vi "FFT滤波无mat程序版.vi"(1 "工频频率":dbl, 2 "样本大小":dbl, 3 "时域波形图":waveform(dbl)[](graph)) -> (0 "时域波形图 2":waveform(dbl)[](graph))   [LabVIEW 2014]
uses:
  <vilib>/Analysis/2dsp.llb/Real FFT.vi
  <vilib>/Analysis/2dsp.llb/Inverse Real FFT.vi
  <vilib>/express/express analysis/Spectral/Block/exnSpectralBlock spectral measurements peak poly.vi
  <vilib>/express/express analysis/Spectral/Block/exnSpectralBlock spectral measurements peak WFM.vi
  <vilib>/express/express analysis/Spectral/XNode/ExpressSpectralMeasurementsBlockNode.xnode
  <vilib>/Analysis/NI_AALPro.lvlib
panel:
  out "时域波形图 3":cluster{"f0":dbl, "df":dbl, "magnitude":dbl[]}(graph)
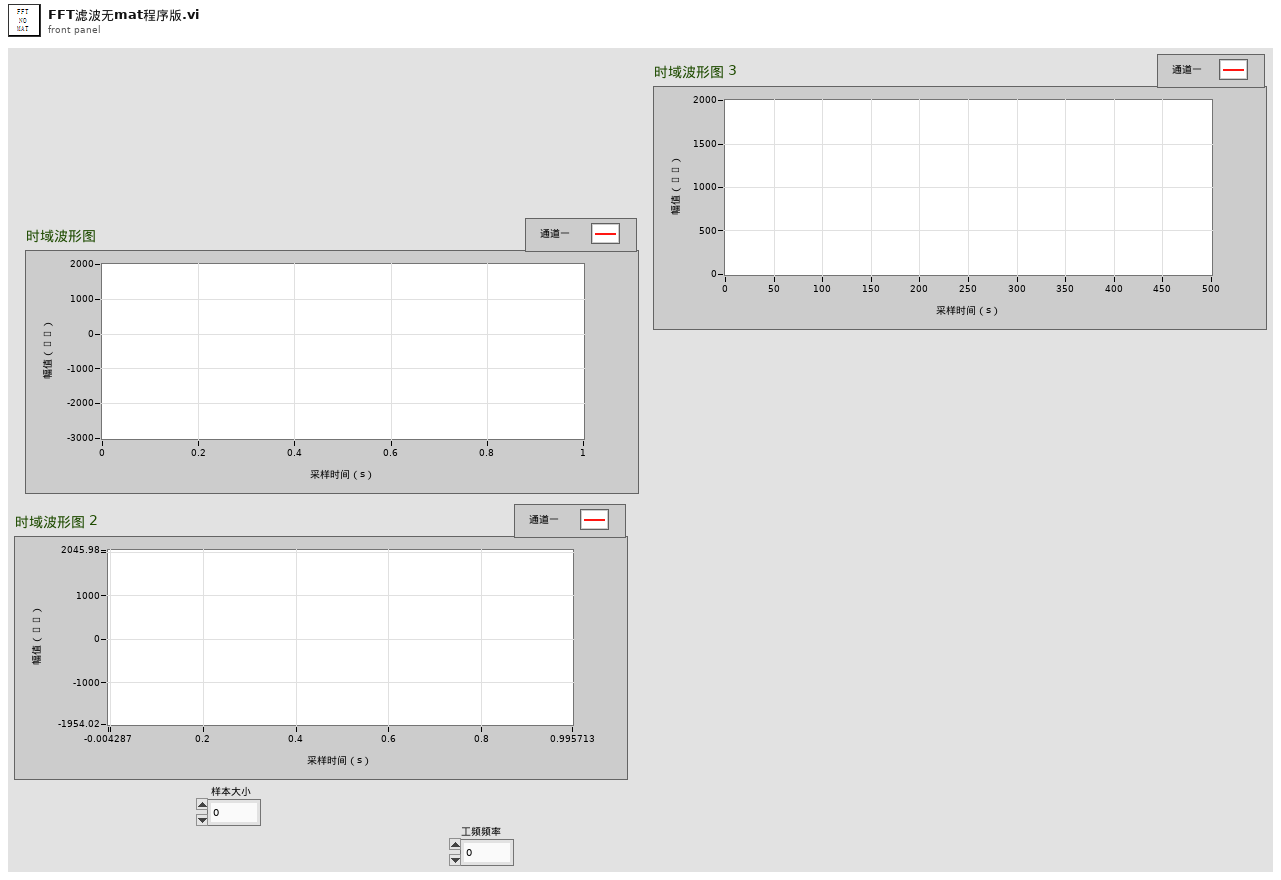
[diagram p1: front panel]
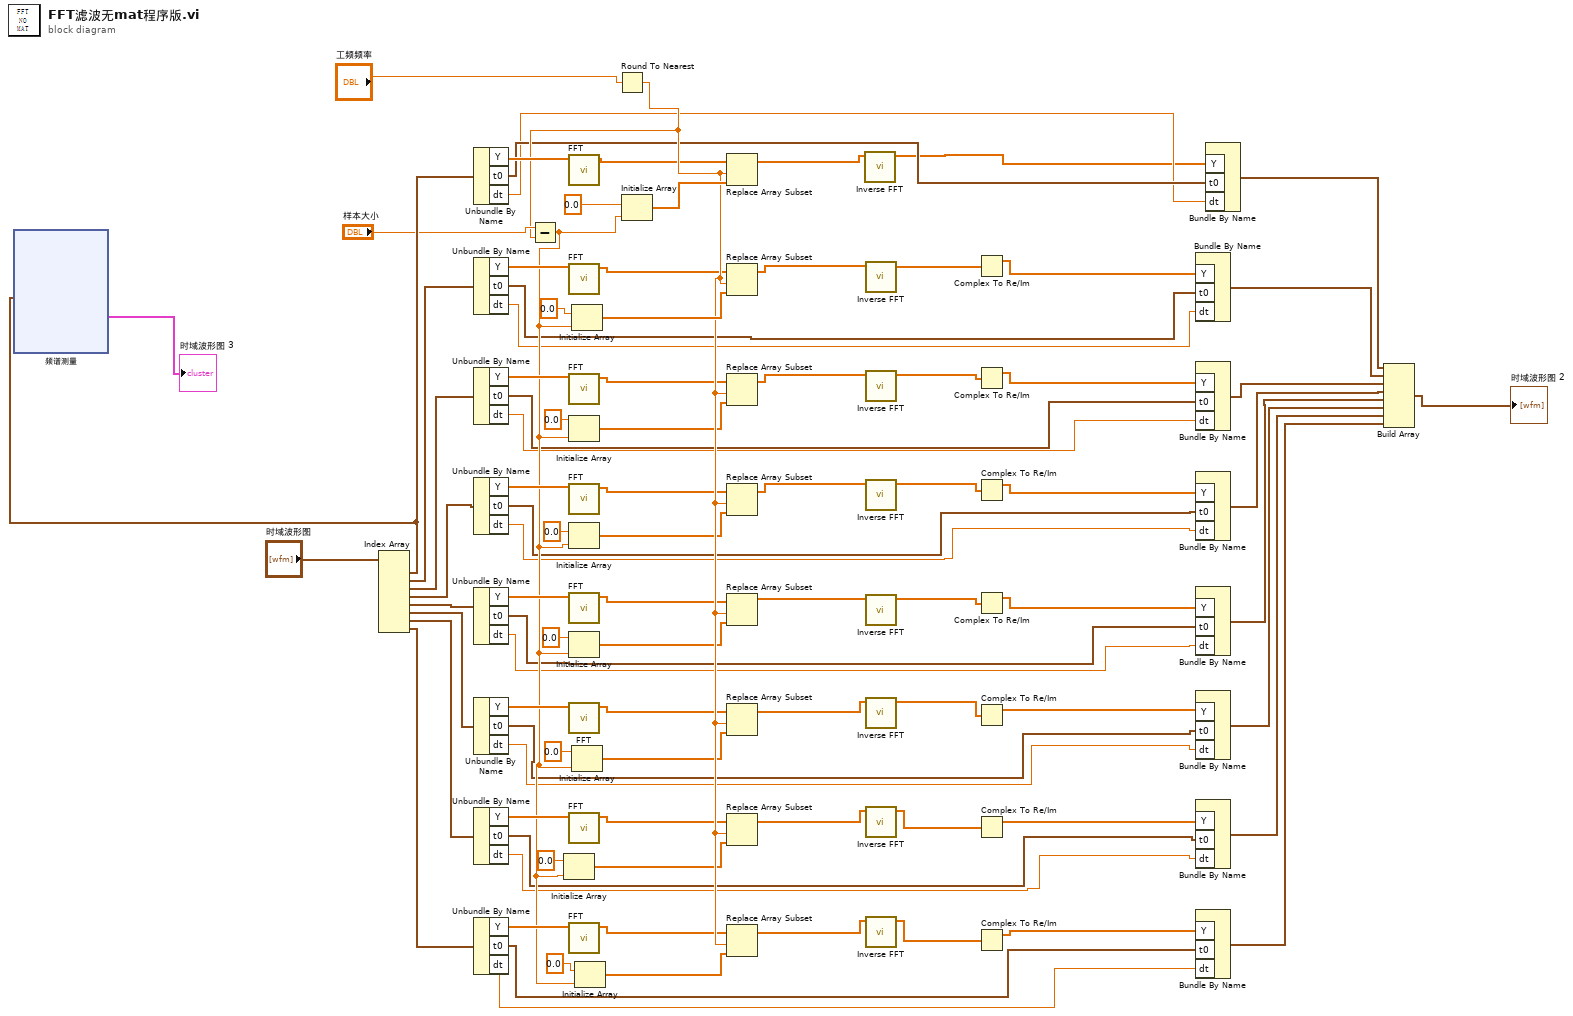
[diagram p0: block diagram]
diagram:
  n1 = Index Array(array="时域波形图") -> (element #1=w70:waveform(dbl), element #2=w93:waveform(dbl), element #3=w92:waveform(dbl), element #4=w91:waveform(dbl), element #5=w90:waveform(dbl), element #6=w89:waveform(dbl), element #7=w88:waveform(dbl), element #8=w87:waveform(dbl))  [unwired: 8 in]
  n2 = xnode "频谱测量"("信号"=w70) -> ("FFT - （峰值）"=→"时域波形图 3":cluster{"f0":dbl, "df":dbl, "magnitude":dbl[]})  [unwired: 1 in, 2 out]
  n3 = Unbundle By Name(w70) -> ("Y"=w86:dbl[], "t0"=w27:timestamp, "dt"=w26:dbl)
  n4 = Unbundle By Name(w93) -> ("Y"=w84:dbl[], "t0"=w25:timestamp, "dt"=w24:dbl)
  n5 = Unbundle By Name(w92) -> ("Y"=w83:dbl[], "t0"=w23:timestamp, "dt"=w22:dbl)
  n6 = Unbundle By Name(w91) -> ("Y"=w82:dbl[], "t0"=w21:timestamp, "dt"=w20:dbl)
  n7 = Unbundle By Name(w90) -> ("Y"=w81:dbl[], "t0"=w19:timestamp, "dt"=w18:dbl)
  n8 = Unbundle By Name(w89) -> ("Y"=w80:dbl[], "t0"=w17:timestamp, "dt"=w16:dbl)
  n9 = Unbundle By Name(w88) -> ("Y"=w79:dbl[], "t0"=w14:timestamp, "dt"=w13:dbl)
  n10 = Unbundle By Name(w87) -> ("Y"=w85:dbl[], "t0"=w12:timestamp, "dt"=w11:dbl)
  n11 = call-poly <vilib>:"FFT.vi"("X"=w86) -> ("FFT {X}"=w10:cdb[])  [unwired: 9 in, 1 out]
  n12 = call-poly <vilib>:"FFT.vi"("X"=w84) -> ("FFT {X}"=w9:cdb[])  [unwired: 9 in, 1 out]
  n13 = call-poly <vilib>:"FFT.vi"("X"=w83) -> ("FFT {X}"=w7:cdb[])  [unwired: 9 in, 1 out]
  n14 = call-poly <vilib>:"FFT.vi"("X"=w82) -> ("FFT {X}"=w6:cdb[])  [unwired: 9 in, 1 out]
  n15 = call-poly <vilib>:"FFT.vi"("X"=w81) -> ("FFT {X}"=w5:cdb[])  [unwired: 9 in, 1 out]
  n16 = call-poly <vilib>:"FFT.vi"("X"=w80) -> ("FFT {X}"=w4:cdb[])  [unwired: 9 in, 1 out]
  n17 = call-poly <vilib>:"FFT.vi"("X"=w79) -> ("FFT {X}"=w3:cdb[])  [unwired: 9 in, 1 out]
  n18 = call-poly <vilib>:"FFT.vi"("X"=w85) -> ("FFT {X}"=w2:cdb[])  [unwired: 9 in, 1 out]
  n19 = Round To Nearest(number="工频频率") -> (nearest integer value=w55:dbl)
  n20 = Subtract(x="样本大小", y=w55) -> (x-y=w57:dbl)
  n21 = Initialize Array(0.0, w57) -> (w50:dbl[])
  n22 = Initialize Array(0.0, w57) -> (w54:dbl[])
  n23 = Initialize Array(0.0, w57) -> (w53:dbl[])
  n24 = Initialize Array(0.0, w57) -> (w52:dbl[])
  n25 = Initialize Array(0.0, w57) -> (w56:dbl[])
  n26 = Initialize Array(0.0, w57) -> (w51:dbl[])
  n27 = Initialize Array(0.0, w57) -> (w49:dbl[])
  n28 = Initialize Array(0.0, w57) -> (w67:dbl[])
  n29 = Replace Array Subset(array=w10, new element=w67, index=w55) -> (w65:cdb[])
  n30 = Replace Array Subset(array=w9, new element=w56, index=w55) -> (w35:cdb[])
  n31 = Replace Array Subset(array=w7, new element=w54, index=w55) -> (w36:cdb[])
  n32 = Replace Array Subset(array=w6, new element=w53, index=w55) -> (w37:cdb[])
  n33 = Replace Array Subset(array=w5, new element=w52, index=w55) -> (w38:cdb[])
  n34 = Replace Array Subset(array=w4, new element=w51, index=w55) -> (w39:cdb[])
  n35 = Replace Array Subset(array=w3, new element=w50, index=w55) -> (w40:cdb[])
  n36 = Replace Array Subset(array=w2, new element=w49, index=w55) -> (w41:cdb[])
  n37 = call-poly <vilib>:"Inverse FFT.vi"("FFT {X}"=w65) -> ("X"=w8:dbl[])  [unwired: 9 in, 1 out]
  n38 = call-poly <vilib>:"Inverse FFT.vi"("FFT {X}"=w35) -> ("X"=w48:dbl[])  [unwired: 9 in, 1 out]
  n39 = call-poly <vilib>:"Inverse FFT.vi"("FFT {X}"=w36) -> ("X"=w47:dbl[])  [unwired: 9 in, 1 out]
  n40 = call-poly <vilib>:"Inverse FFT.vi"("FFT {X}"=w37) -> ("X"=w46:dbl[])  [unwired: 9 in, 1 out]
  n41 = call-poly <vilib>:"Inverse FFT.vi"("FFT {X}"=w38) -> ("X"=w45:dbl[])  [unwired: 9 in, 1 out]
  n42 = call-poly <vilib>:"Inverse FFT.vi"("FFT {X}"=w39) -> ("X"=w44:dbl[])  [unwired: 9 in, 1 out]
  n43 = call-poly <vilib>:"Inverse FFT.vi"("FFT {X}"=w40) -> ("X"=w43:dbl[])  [unwired: 9 in, 1 out]
  n44 = call-poly <vilib>:"Inverse FFT.vi"("FFT {X}"=w41) -> ("X"=w42:dbl[])  [unwired: 9 in, 1 out]
  n45 = Complex To Re/Im(x + iy=w48) -> (x=w34:dbl[])  [unwired: 1 out]
  n46 = Complex To Re/Im(x + iy=w47) -> (x=w33:dbl[])  [unwired: 1 out]
  n47 = Complex To Re/Im(x + iy=w46) -> (x=w32:dbl[])  [unwired: 1 out]
  n48 = Complex To Re/Im(x + iy=w45) -> (x=w31:dbl[])  [unwired: 1 out]
  n49 = Complex To Re/Im(x + iy=w44) -> (x=w30:dbl[])  [unwired: 1 out]
  n50 = Complex To Re/Im(x + iy=w43) -> (x=w29:dbl[])  [unwired: 1 out]
  n51 = Complex To Re/Im(x + iy=w42) -> (x=w28:dbl[])  [unwired: 1 out]
  n52 = Bundle By Name("Y"=w34, "t0"=w25, "dt"=w24) -> (w77:waveform(dbl))  [unwired: 1 in]
  n53 = Bundle By Name("Y"=w33, "t0"=w23, "dt"=w22) -> (w76:waveform(dbl))  [unwired: 1 in]
  n54 = Bundle By Name("Y"=w32, "t0"=w21, "dt"=w20) -> (w75:waveform(dbl))  [unwired: 1 in]
  n55 = Bundle By Name("Y"=w31, "t0"=w19, "dt"=w18) -> (w74:waveform(dbl))  [unwired: 1 in]
  n56 = Bundle By Name("Y"=w30, "t0"=w17, "dt"=w16) -> (w73:waveform(dbl))  [unwired: 1 in]
  n57 = Bundle By Name("Y"=w29, "t0"=w14, "dt"=w13) -> (w15:waveform(dbl))  [unwired: 1 in]
  n58 = Bundle By Name("Y"=w28, "t0"=w12, "dt"=w11) -> (w72:waveform(dbl))  [unwired: 1 in]
  n59 = Bundle By Name("Y"=w8, "t0"=w27, "dt"=w26) -> (w78:waveform(dbl))  [unwired: 1 in]
  n60 = Build Array(w78, w77, w76, w75, w74, w73, w15, w72) -> (→"时域波形图 2":waveform(dbl)[])
